vi "Database Command Parameters Refresh.vi"(8 "error in (no error)":errorcluster caption="错误输入（无错误）", 11 "Database Command 输入":refnum<class "Database Command.lvclass"> caption="DNL_LabVIEW Object in") -> (0 "error out":errorcluster caption="错误输出", 3 "Database Command 输出":refnum<class "Database Command.lvclass"> caption="DNL_LabVIEW Object out")   [LabVIEW 2011, in "Database Command.lvclass"]
uses:
  Database Command.lvclass
  Database Command.lvclass/Database Command.ctl
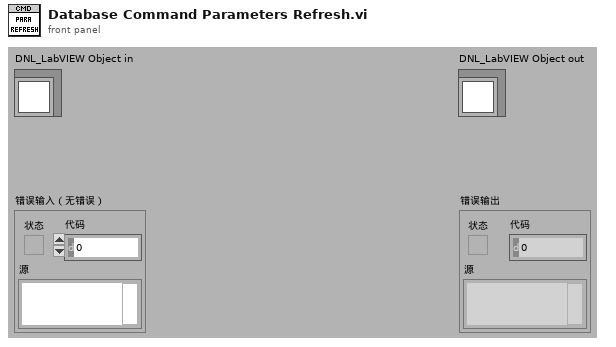
[diagram p1: front panel]
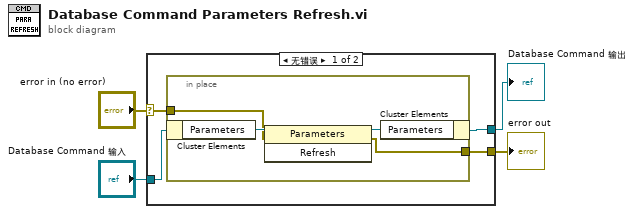
[diagram p0: block diagram]
diagram:
  n1 = case shown="无错误" "error in (no error)" {
    selector: "error in (no error)" -> [w6 w14]
    tunnel: [w5 w14] -> w3
    tunnel: [w7 w13] -> w1
    tunnel: "Database Command 输入" -> [w8 w13]
    frame No Error {
      n2 = in-place {
        in-place-border: w6 -> [w10]
        in-place-border: [w9] -> w5
        n3 = in-place-cluster #1(w8) -> ("Parameters"=w12:refnum<k7>)
        n4 = invoke class="Parameters" method="Refresh"(reference=w12, error in=w10) -> (reference out=w11:refnum<k7>, error out=w9:errorcluster)  [unwired: 1 in, 1 out]
        n5 = in-place-cluster #1("Parameters"=w11) -> (w7:refnum<class "Database Command.lvclass">)
      }
    }
    frame Error {
    }
  }
  "error out" <- w3
  "Database Command 输出" <- w1
